vi "find_interference_cornea.vi"(8 "干涉长度":i32=50, 9 "阈值":dbl=2.2, 10 "A":dbl[](array[numeric])=array[267857 elements], 11 "S":dbl[](array[numeric])=array[267857 elements]) -> (1 "Max_Index":i32, 2 "个数":u32=2, 3 "INDEX":i32[](array[numeric]))   [LabVIEW 2015, in "Boimetry Processing.lvlib"]
uses:
  Boimetry Processing.lvlib
  <vilib>/Analysis/NI_AALPro.lvlib
  <vilib>/Analysis/NI_AAL_SigProc.lvlib
panel:
  out "x-y":dbl[](array[numeric])
  out "数组":dbl[](array[numeric])
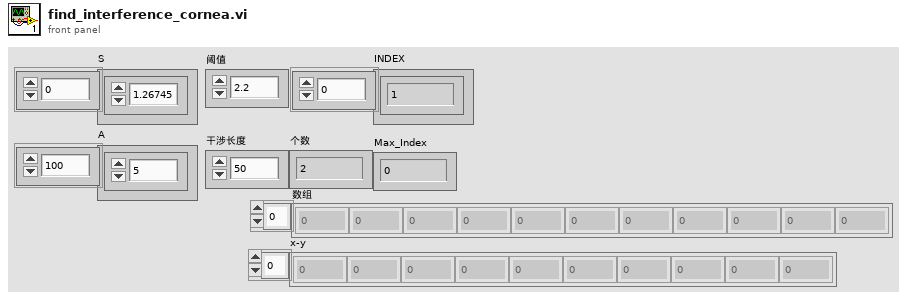
[diagram p1: front panel]
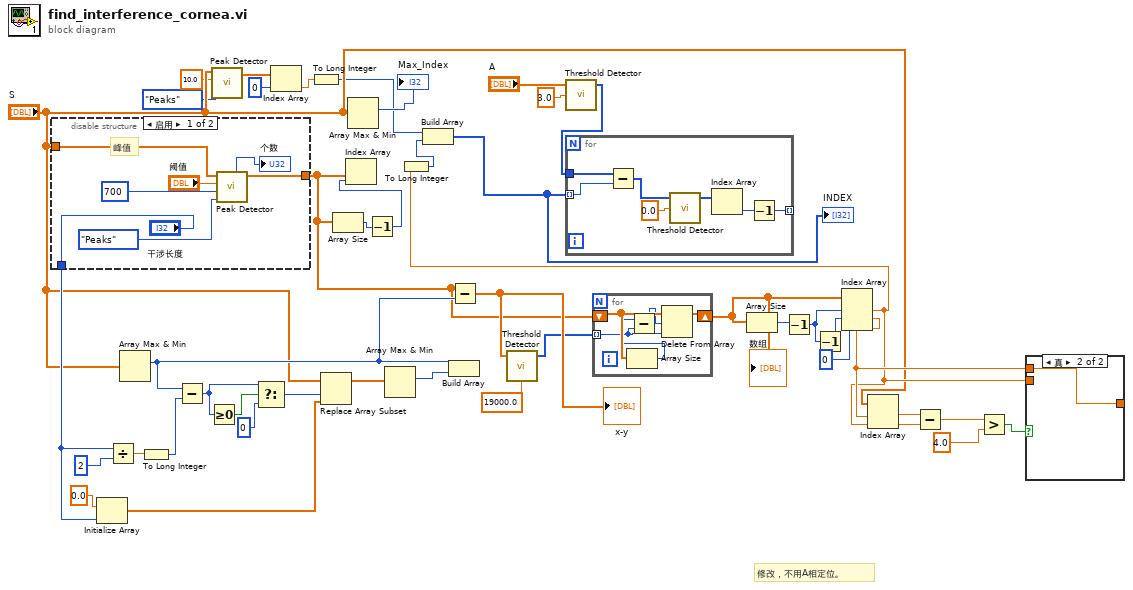
[diagram p0: block diagram]
diagram:
  # "修改，不用A相定位。"
  n1 = disable-structure shown="启用" {
    disable-tunnel: "S" -> [w51 _]
    disable-tunnel: [w47 _] -> w13
    disable-tunnel: ["干涉长度" _] -> w28
    frame Enabled {
      # "峰值"
      n2 = call <vilib>:"Peak Detector.vi"("peaks/valleys"=enum32{"Peaks", "Valleys"}."Peaks", "width"=700, "threshold"="阈值", "X"=w51) -> ("Locations"=w47:dbl[], "# found"=→"个数":i32)  [unwired: 3 in, 3 out]
    }
    frame Disabled {
    }
  }
  n3 = Initialize Array(0.0 ("元素"), w28) -> (w29:dbl[])
  n4 = Divide(x=w28, y=u32 2) -> (x/y=w38:dbl)
  n5 = Array Max & Min(array="S") -> (max index (indices)=w27:i32)  [unwired: 3 out]
  n6 = To Long Integer(number=w38) -> (32bit integer=w37:i32)
  n7 = Subtract(x=w27, y=w37) -> (x-y=w33:i32)
  n8 = Greater Or Equal To 0?(x=w33) -> (x >= 0?=w34:bool)
  n9 = call <vilib>:"Peak Detector.vi"("peaks/valleys"=enum32{"Peaks", "Valleys"}."Peaks", "threshold"=10.0, "X"="S") -> ("Locations"=w5:dbl[])  [unwired: 4 in, 4 out]
  n10 = Select(t=w33, s=w34, f=u32 0) -> (s? t:f=w31:u32)
  n11 = Index Array(array=w5, index=0 ("索引")) -> (element=w3:dbl)
  n12 = To Long Integer(number=w3) -> (32bit integer=w2:i32)
  n13 = Replace Array Subset(array="S", new element=w29, index=w31) -> (w30:dbl[])
  n14 = Array Size(array=w13) -> (size(s)=w42:i32)
  n15 = Array Max & Min(array="S") -> (max index (indices)=→"Max_Index":i32)  [unwired: 3 out]
  n16 = Decrement(x=w42) -> (x-1=w41:i32)
  n17 = Index Array(array=w13, index=w41) -> ()  [unwired: 1 out]
  n18 = Array Max & Min(array=w30) -> (max index (indices)=w35:i32)  [unwired: 3 out]
  n19 = Build Array(w27, w35) -> ()  [unwired: 1 out]
  n20 = Subtract(x=w13, y=w27) -> (x-y=w26:dbl[])
  "x-y" <- w26
  n21 = call <vilib>:"Threshold Detector.vi"("threshold"=19000.0, "X"=w26) -> ("Indices"=w24:i32[])  [unwired: 1 in, 2 out]
  n22 = call <vilib>:"Threshold Detector.vi"("threshold"=3.0, "X"="A") -> ("Indices"=w40:i32[])  [unwired: 1 in, 2 out]
  n23 = for {
    tunnel: w24 -> [w52] mode=indexing
    shift-right: [w56] -> w23
    shift-left: w13 -> [w55]
    n24 = Array Size(array=w55) -> (size(s)=w53:i32)
    n25 = Subtract(x=w53, y=w52) -> (x-y=w54:i32)
    n26 = Delete From Array(array=w55, length=w54, index=w52) -> (array with subset deleted=w56:dbl[])  [unwired: 1 out]
  }
  "数组" <- w23
  n27 = Array Size(array=w23) -> (size(s)=w22:i32)
  n28 = Decrement(x=w22) -> (x-1=w21:i32)
  n29 = Decrement(x=w21) -> (x-1=w20:i32)
  n30 = Index Array(array=w23, index #1=w21, index #2=w20, index #3=0 ("索引")) -> (element #1=w9:dbl, element #2=w14:dbl)  [unwired: 1 out]
  n31 = To Long Integer(number=w9) -> (32bit integer=w10:i32)
  n32 = Build Array(w2, w10) -> (w1:i32[])
  "INDEX" <- w1
  n33 = for {
    tunnel: w1 -> [w63] mode=indexing
    tunnel: w40 -> [w59]
    tunnel: [w57] -> _ mode=indexing
    n34 = Subtract(x=w59, y=w63) -> (x-y=w61:i32[])
    n35 = call <vilib>:"Threshold Detector.vi"("threshold"=0.0, "X"=w61) -> ("Indices"=w60:i32[])  [unwired: 1 in, 2 out]
    n36 = Index Array(array=w60) -> (element=w58:i32)  [unwired: 1 in]
    n37 = Decrement(x=w58) -> (x-1=w57:i32)
  }
  n38 = Index Array(array="S", index #1=w14, index #2=w9) -> (element #1=w18:dbl, element #2=w19:dbl)
  n39 = Subtract(x=w18, y=w19) -> (x-y=w15:dbl)
  n40 = Greater?(x=w15, y=4.0) -> (0:w16:bool)
  n41 = case shown="真" w16 {
    tunnel: [w64 w65] -> _
    tunnel: w14 -> [_ w65]
    tunnel: w9 -> [w64 _]
    frame False {
    }
    frame True {
    }
  }
